vi "1,3 B Spoof Reality.vi"(9 "Robot Initial Position\nFrom Simulator SW corner":T1={"East"=20.0, "North"=20.0}, 11 "Simulator Bounds":T3={"Simulator E Range"=20.0, "Simulator E Min"=-10.0, "Simulator N Range"=20.0, "Simulator N Min"=-10.0}) -> (0 "Apparent Wind\nDirection":T6, 1 "Apparent Wind\nSpeed":T4, 2 "Robot velocity":T2 {"East" format="%#_5g"}, 3 "Robot\nHeading":T5 format="%05.1f", 4 "Boat Path":cluster{"X Position":dbl, "Y Position":dbl}[](array[cluster]), 5 "Robot UTM Location":T7 {"North" format="%#_10f"; "East" format="%#_8f"}, 6 "XY Graph":cluster{dbl, dbl}[](graph))   [LabVIEW 2011]
uses:
  2-Think/2 Typedefs/UTM Location.ctl
  2-Think/2 Typedefs/heading.ctl
  2-Think/2 Typedefs/apparent wind direction.ctl
  2-Think/2 Typedefs/apparent wind speed.ctl
  2-Think/2 Typedefs/Velocity.ctl
  1,3 B Typedefs/simulator bounds.ctl
  2-Think/2 Typedefs/robot velocity.ctl
  2-Think/2 Typedefs/rate of turn.ctl
  2-Think/2 Typedefs/pitch and roll.ctl
  2-Think/2 Typedefs/generalized sensor status.ctl
  2-Think/2 Typedefs/indicator LED.ctl
  2-Think/2 Typedefs/generalized actuator status.ctl
  2-Think/2 Globals/2 Global.vi
panel:
  in  "Absolute Water Current":T2 {"East" format="%#_5g"}
  out "Wind dV":T4
  out "Total Drag dV":dbl
  out "Rudder Drag":dbl
  in  "Rudder Drag Coefficient":dbl=1.5
  out "Speed":T4
  in  "Hull Drag Coefficient":dbl=0.3
  out "dHeading/dT":T5 format="%05.1f"
  out "Apparent Wind":cluster{"X Position":dbl, "Y Position":dbl}
  in  "Wind Direction":dbl=45.0
  in  "Wind Speed":dbl=2.0
  # "Add reasonable values to all of the things you can set here."
  # "This is the Bass. It's catchy. You like it."
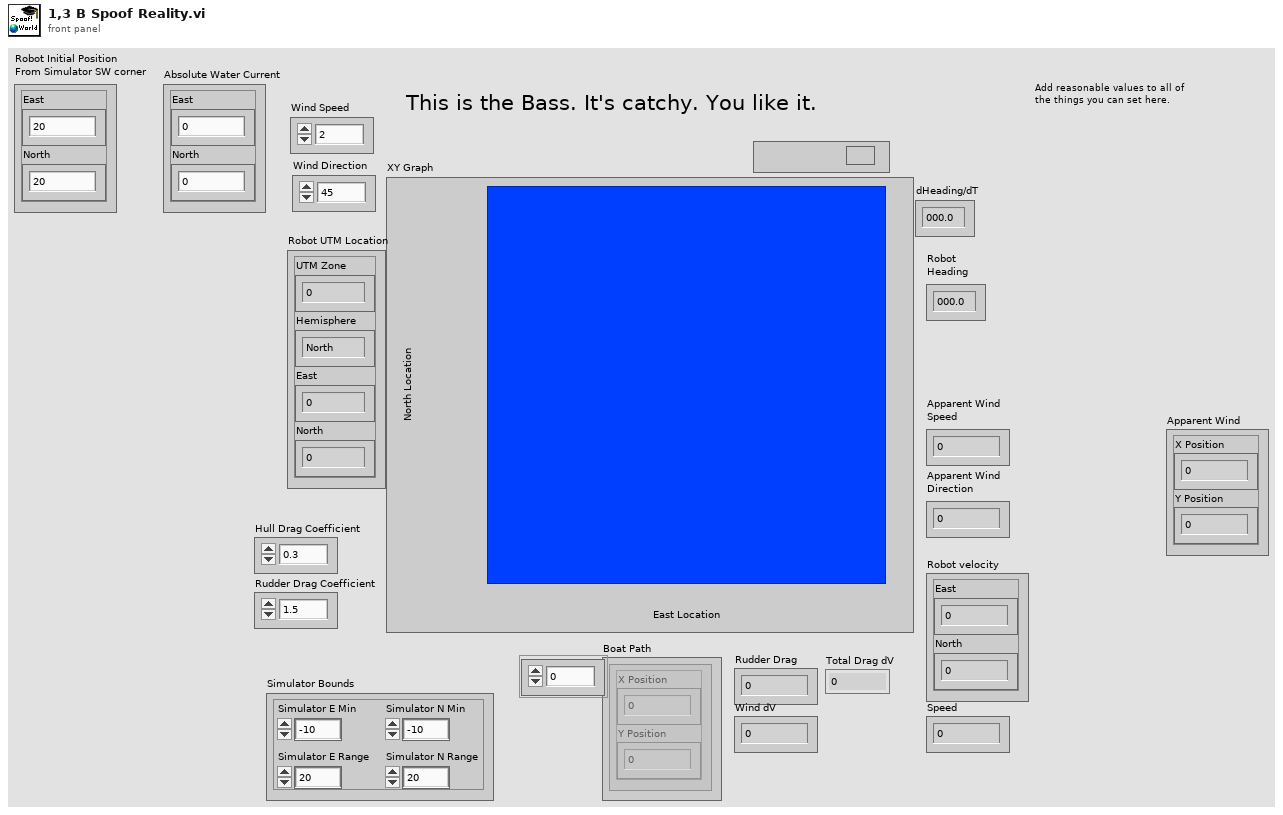
[diagram p1: front panel]
types:
  T1 = typedef "robot velocity.ctl" = cluster{"East":dbl, "North":dbl}
  T2 = typedef "Velocity.ctl" = cluster{"East":dbl, "North":dbl}
  T3 = typedef "simulator bounds.ctl" = cluster{"Simulator E Range":dbl, "Simulator E Min":dbl, "Simulator N Range":dbl, "Simulator N Min":dbl}
  T4 = typedef "apparent wind speed.ctl" = dbl
  T5 = typedef "heading.ctl" = dbl
  T6 = typedef "apparent wind direction.ctl" = dbl
  T7 = typedef "UTM Location.ctl" = cluster{"UTM Zone":dbl, "Hemisphere":enum16{"North", "South"}, "East":dbl, "North":dbl}
  T8 = typedef "rate of turn.ctl" = dbl
  T9 = typedef "pitch and roll.ctl" = cluster{"Pitch":dbl, "Roll":dbl}
  T10 = typedef "generalized sensor status.ctl" = cluster{"Sensor Connected":T11, "Sensor Initialized":T11, "Sensor OK":T11, "Latest Error String":string, "GPS Lock":T11}
  T11 = typedef "indicator LED.ctl" = bool
  T12 = typedef "generalized actuator status.ctl" = cluster{"Actuator Connected":T11}
  T13 = typedef "apparent wind.ctl" = cluster{"Toward Fore":dbl, "Toward Starboard":dbl}
  T14 = typedef "setpoints to boat.ctl" = cluster{"Sail Position":T15, "Rudder Angle":T16}
  T15 = typedef "sail setpt.ctl" = dbl
  T16 = typedef "rudder angle.ctl" = dbl
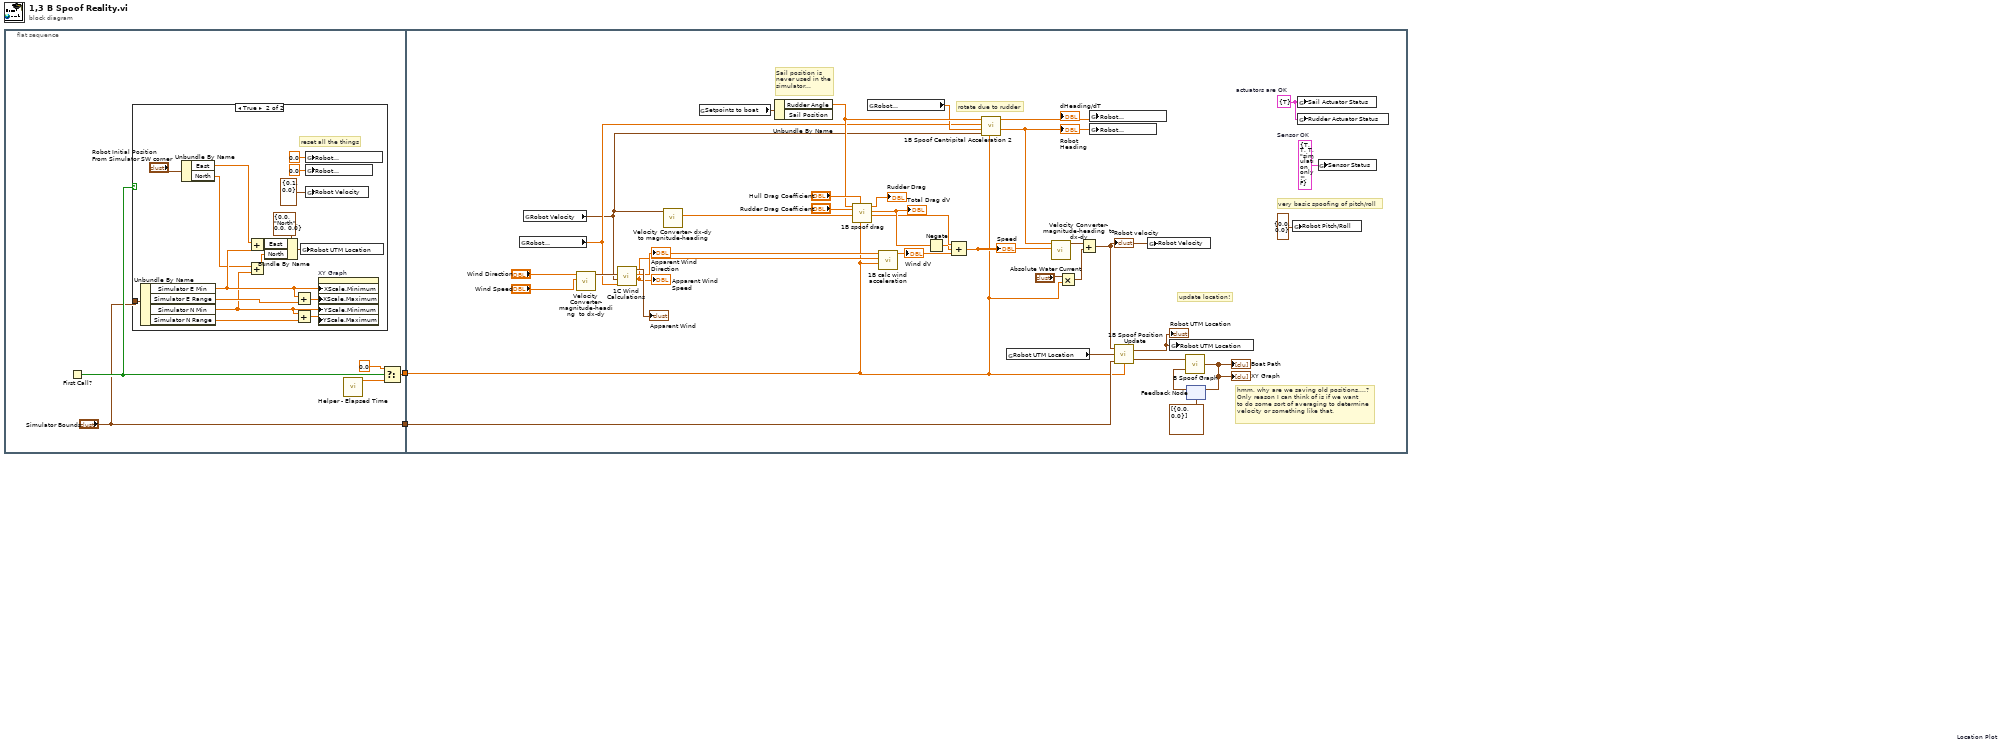
[diagram p0: block diagram]
diagram:
  n1 = flat-sequence {
    tunnel: [w7] -> w2
    tunnel: ["Simulator Bounds"] -> w1
    tunnel: w2 -> [w25]
    tunnel: w1 -> [w30]
    frame #0 {
      n2 = First Call?() -> (First Call?: T/F=w6:bool)
      n3 = case shown="True" w6 {
        tunnel: "Simulator Bounds" -> [_ w21]
        frame False {
        }
        frame True {
          # "reset all the things"
          n4 = Unbundle By Name(w21) -> ("Simulator E Min"=w16:dbl, "Simulator E Range"=w15:dbl, "Simulator N Min"=w8:dbl, "Simulator N Range"=w12:dbl)
          n5 = Unbundle By Name("Robot Initial Position\nFrom Simulator SW corner") -> ("East"=w10:dbl, "North"=w9:dbl)
          n6 = Add(x=w10, y=w16) -> (x+y=w14:dbl)
          n7 = Add(x=w9, y=w8) -> (x+y=w13:dbl)
          n8 = Bundle By Name(cluster=T7 {"UTM Zone"=0.0, "Hemisphere"=enum."North", "East"=0.0, "North"=0.0} ("Robot UTM Location"), "East"=w14, "North"=w13) -> (w18:T7)
          n9 = Add(x=w16, y=w15) -> (x+y=w20:dbl)
          n10 = Add(x=w8, y=w12) -> (x+y=w19:dbl)
          n11 = global write "2 Global.vi" "Robot UTM Location"(w18) -> ()
          n12 = global write "2 Global.vi" "Robot\nRate of Turn"(T8 0.0 ("Robot\nRate of Turn")) -> ()
          n13 = global write "2 Global.vi" "Robot\nHeading"(T5 0.0 ("Robot\nHeading")) -> ()
          n14 = global write "2 Global.vi" "Robot Velocity"(T1 {"East"=0.1, "North"=0.0} ("Robot Velocity")) -> ()
          n15 = property on="XY Graph" class="XYGraph (strict)"("XScale.Minimum"=w16, "XScale.Maximum"=w20, "YScale.Minimum"=w8, "YScale.Maximum"=w19) -> ()  [unwired: 2 in, 2 out]
        }
      }
      n16 = call "Helper - Elapsed Time.vi"() -> ("Time Elapsed (s)\nSince Last Iteration"=w4:dbl)  [unwired: 10 in, 1 out]
      n17 = Select(t=0.0 ("f"), s=w6, f=w4) -> (s? t:f=w7:dbl)
    }
    frame #1 {
      w54 = T10 {"Sensor Connected"=TRUE, "Sensor Initialized"=TRUE, "Sensor OK"=TRUE, "Latest Error String"="simulation only!", "GPS Lock"=FALSE}  # Sensor OK
      w55 = T12 {"Actuator Connected"=TRUE}  # actuators are OK
      # "Sail position is never used in the simulator..."
      # "hmm, why are we saving old positions....?\nOnly reason I can think of is if we want\nto do some sort of averaging to determine\nvelocity or something like that."
      # "rotate due to rudder"
      # "update location!"
      # "very basic spoofing of pitch/roll"
      n18 = global read "2 Global.vi" "Robot\nHeading"() -> (w34:T5)
      n19 = global read "2 Global.vi" "Robot Velocity"() -> (w33:T1)
      n20 = call "Velocity Converter- magnitude-heading  to dx-dy.vi"("Magnitude"="Wind Speed", "Heading"="Wind Direction") -> ("Vector Out"=w51:T2)  [unwired: 9 in]
      n21 = call "1C Wind Calculations.vi"("Boat Heading"=w34, "Boat Velocity"=w33, "Absolute Wind"=w51) -> ("Apparent Wind Speed"=w46:T4, "Apparent Wind\nDirection"=w47:T6, "Apparent Wind"=→"Apparent Wind":T13)  [unwired: 5 in]
      "Apparent Wind\nDirection" <- w47
      "Apparent Wind\nSpeed" <- w46
      n22 = call "Velocity Converter- dx-dy to magnitude-heading.vi"("Vector In"=w33) -> ("Magnitude Out"=w38:dbl)  [unwired: 9 in, 1 out]
      n23 = global read "2 Global.vi" "Setpoints to boat"() -> (w56:T14)
      n24 = Unbundle By Name(w56) -> ("Rudder Angle"=w42:T16)  [unwired: 1 out]
      n25 = call "1B spoof drag.vi"("time elapsed since last iteration"=w25, "Hull Drag Coefficient"="Hull Drag Coefficient", "Speed"=w38, "Rudder Drag Coefficient"="Rudder Drag Coefficient", "Rudder Angle"=w42) -> ("Total Drag dV"=w39:dbl, "Rudder Drag"=→"Rudder Drag":dbl)  [unwired: 5 in]
      "Total Drag dV" <- w39
      n26 = global read "2 Global.vi" "Robot\nRate of Turn"() -> (w35:T8)
      n27 = call "1B calc wind acceleration.vi"("time elapsed since last iteration"=w25, "Apparent Wind Speed in"=w46, "Apparent Wind\nDirection"=w47) -> ("Wind dV"=w36:T4)  [unwired: 8 in]
      "Wind dV" <- w36
      n28 = Negate(x=w39) -> (-x=w37:dbl)
      n29 = Compound Arithmetic op=ADD(w38, w37, w36) -> (w40:T4)
      "Speed" <- w40
      n30 = call "1B Spoof Centripital Acceleration 2.vi"("time elapsed since last iteration"=w25, "Robot Velocity"=w33, "dHeading/dT in"=w35, "Robot\nHeading in"=w34, "Rudder Angle"=w42) -> ("Robot\nHeading out"=w44:T5, "dHeading/dT"=w49:T5)  [unwired: 4 in, 1 out]
      "Robot\nHeading" <- w44
      "dHeading/dT" <- w49
      n31 = global read "2 Global.vi" "Robot UTM Location"() -> (w32:T7)
      n32 = call "Velocity Converter- magnitude-heading  to dx-dy.vi"("Magnitude"=w40, "Heading"=w44) -> ("Vector Out"=w29:T2)  [unwired: 9 in]
      n33 = Multiply(x="Absolute Water Current", y=w25) -> (x*y=w26:T2)
      n34 = Add(x=w29, y=w26) -> (x+y=w28:T2)
      "Robot velocity" <- w28
      n35 = global write "2 Global.vi" "Robot\nRate of Turn"(w49) -> ()
      n36 = global write "2 Global.vi" "Robot\nHeading"(w44) -> ()
      n37 = call "1B Spoof Position Update.vi"("dt"=w25, "Simulator Bounds"=w30, "Robot UTM Location"=w32, "Robot Velocity"=w28) -> ("New Position (X,Y)"=w57:cluster{"X Position":dbl, "Y Position":dbl}, "New Robot UTM Location"=w31:T7)
      "Robot UTM Location" <- w31
      n38 = global write "2 Global.vi" "Robot Velocity"(w28) -> ()
      n39 = global write "2 Global.vi" "Robot UTM Location"(w31) -> ()
      n40 = feedback #1 "Location Plot"(cluster{dbl, dbl}[] [{0.0, 0.0}] ("XY Graph")) -> (w58:cluster{dbl, dbl}[])
      n41 = call "B Spoof Graph.vi"("XY Graph"=w58, "New Position"=w57) -> ("Array"=w59:cluster{"X Position":dbl, "Y Position":dbl}[])
      "XY Graph" <- w59
      "Boat Path" <- w59
      n42 = feedback-in #1(w59) -> ()
      n43 = global write "2 Global.vi" "Robot Pitch/Roll"(T9 {"Pitch"=0.0, "Roll"=0.0} ("Robot Pitch/Roll")) -> ()
      n44 = global write "2 Global.vi" "Sail Actuator Status"(w55) -> ()
      n45 = global write "2 Global.vi" "Rudder Actuator Status"(w55) -> ()
      n46 = global write "2 Global.vi" "Sensor Status"(w54) -> ()
    }
  }
